vi "Obtain Debug Queue.vi"() -> (0 "Debug Queue":T1)   [LabVIEW 2013]
uses:
  Sidecar Debug Queue.ctl
  Experimental Configuration.ctl
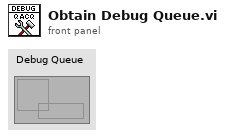
[diagram p1: front panel]
types:
  T1 = typedef "Sidecar Debug Queue.ctl" = refnum<queue>
  T2 = typedef "Experimental Configuration.ctl" = cluster{"Output Waveforms":waveform(dbl)[], "Output Channels":string, "Input Channels":string, "DAQ Data Notifier Name":string}
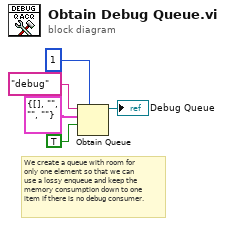
[diagram p0: block diagram]
diagram:
  # "We create a queue with room for\nonly one element so that we can\nuse a lossy enqueue and keep the\nmemory consumption down to one\nitem if there is no debug consumer."
  n1 = Obtain Queue(max queue size (-1, unlimited)=1, name (unnamed)="debug", element data type=T2 {"Output Waveforms"=[], "Output Channels"="", "Input Channels"="", "DAQ Data Notifier Name"=""} ("Experimental Configuration"), create if not found? (T)=TRUE) -> (queue out=→"Debug Queue":refnum<queue>)  [unwired: 1 in, 2 out]
